vi "TestTimingGrip.vi"() -> ()   [LabVIEW 2017]
uses:
  Projekt-RubikLibrary/ServoEnumControl.ctl
  <vilib>/myRIO/Common/Instrument Driver Framework/myRIO v1.0/UART/vis/myRIO v1.0 Close UART.vi
  <vilib>/myRIO/Common/Instrument Driver Framework/Utilities/vis/FPGA Ref Manager.vi
  <vilib>/myRIO/Common/Instrument Driver Framework/myRIO v1.0/myRIO v1.0 Reset FPGA.vi
  <vilib>/myRIO/Common/Instrument Driver Framework/myRIO v1.0/IRQ/vis/myRIO v1.0 IRQ Info FGV.vi
  <vilib>/myRIO/Common/Instrument Driver Framework/myRIO v1.0/IRQ/vis/myRIO v1.0 Timer IRQ Info FGV.vi
  <vilib>/myRIO/Common/Instrument Driver Framework/myRIO v1.0/IRQ/vis/myRIO v1.0 ISR Agent.vi
  Projekt-RubikLibrary/RubikLibrary.lvlib
  <vilib>/myRIO/Instrument Drivers/Utilities/Utilities.lvlib
  Projekt-RubikLibrary/RubikLibraryRT.lvlib
panel:
  in  "milliseconds to wait":u32=500
  in  "Start":bool
  in  "Number of loops":i32=5
  in  "stop":bool
  # "TestTimingTurn"
  # "Initial positions:\nFront servo open and 0°\nLeft and right servo 0°"
  # "Is 90° reached and a small delay?"
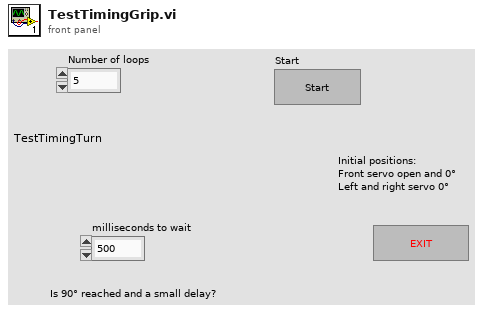
[diagram p1: front panel]
types:
  T1 = typedef "RubikLibrary.lvlib/ServoEnumControl.ctl" = enum16{"Left Servo", "Front Servo", "Right Servo"}
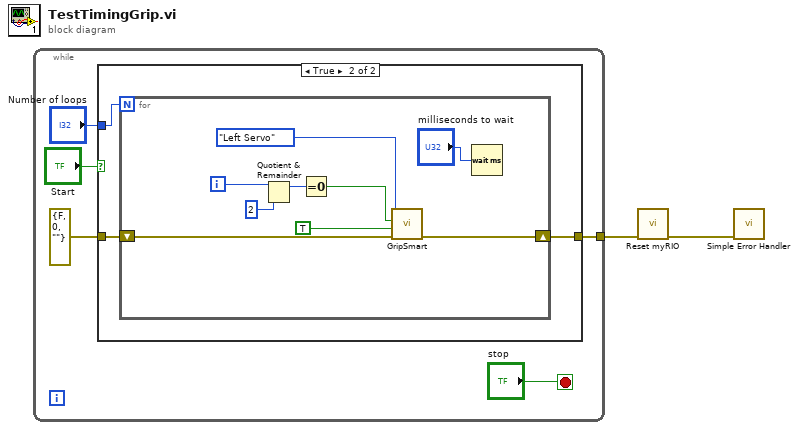
[diagram p0: block diagram]
diagram:
  n1 = while {
    tunnel: [w6] -> w2
    stop <- "stop" stop-if-true
    n2 = case shown="True" "Start" {
      tunnel: [w8 w11] -> w6
      tunnel: errorcluster {"status"=FALSE, "code"=0, "source"=""} ("error in") -> [w8 w10]
      tunnel: "Number of loops" -> [_ w9]
      frame False {
      }
      frame True {
        n3 = for {
          N: w9 -> [_]
          shift-right: [w16] -> w11
          shift-left: w10 -> [w15]
          i -> [w20]
          n4 = Quotient & Remainder(x=w20, y=2) -> (x-y*floor(x/y)=w18:i32)  [unwired: 1 out]
          n5 = Equal To 0?(x=w18) -> (x = 0?=w12:bool)
          n6 = call "GripSmart.vi"("error in"=w15, "NoWait"=TRUE, "Grip closed (in)"=w12, "Servo"=ServoEnumControl."Left Servo") -> ("error out"=w16:errorcluster)  [unwired: 6 in, 1 out]
          n7 = Wait (ms)(milliseconds to wait="milliseconds to wait") -> ()  [unwired: 1 out]
        }
      }
    }
  }
  n8 = call <vilib>:"Reset myRIO.vi"("error in (no error)"=w2) -> ("error out"=w1:errorcluster)  [unwired: 10 in]
  n9 = call <vilib>:"Simple Error Handler.vi"("error in (no error)"=w1) -> ()  [unwired: 4 in, 5 out]
